vi "Konvolucio MCAN120803 Example_0005 WriteSingleFrame.vi"   [LabVIEW 2011]
uses:
  <instrlib>/Konvolucio MCAN120803/Public/Attributes/AttrSetTermination.vi
  <instrlib>/Konvolucio MCAN120803/Konvolucio MCAN120803.lvlib
types:
  T1 = typedef "Konvolucio MCAN120803.lvlib/CanHandleType.ctl" = cluster{"AdapterDevice":refnum<k24>}
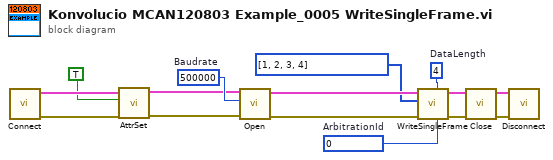
[diagram p0: block diagram]
diagram:
  w1 = u32 0  # ArbitrationId
  w3 = u8 4  # DataLength
  w15 = u32 500000  # Baudrate
  n1 = call <instrlib>:"Connect.vi"() -> ("error out"=w12:errorcluster, "CanHandleOut"=w10:T1)  [unwired: 10 in]
  n2 = call-poly <instrlib>:"AttrSet.vi"("error in"=w12, "Enabled"=TRUE, "CanHandleIn"=w10) -> ("error out"=w11:errorcluster, "CanHandleOut"=w9:T1)  [unwired: 6 in]
  n3 = call <instrlib>:"Open.vi"("error in"=w11, "Baudrate"=w15, "CanHandleIn"=w9) -> ("error out"=w14:errorcluster, "CanHandleOut"=w13:T1)  [unwired: 7 in]
  n4 = call <instrlib>:"WriteSingleFrame.vi"("ArbitrationId"=w1, "DataLength"=w3, "error in"=w14, "Data"=u8[] [1, 2, 3, 4], "CanHandleIn"=w13) -> ("error out"=w7:errorcluster, "CanHandleOut"=w6:T1)  [unwired: 5 in]
  n5 = call <instrlib>:"Close.vi"("error in"=w7, "CanHandleIn"=w6) -> ("error out"=w5:errorcluster, "CanHandleOut"=w4:T1)  [unwired: 8 in]
  n6 = call <instrlib>:"Disconnect.vi"("error in"=w5, "CanHandleIn"=w4) -> ()  [unwired: 9 in, 1 out]
